vi "signal_mapping_PMT-measurement_7_9.vi"() -> ()   [LabVIEW 2024]
uses:
  <vilib>/Analysis/1siggen.llb/Ramp Pattern by Samples.vi
  <vilib>/Utility/file.llb/Write Delimited Spreadsheet (string).vi
  <vilib>/Utility/file.llb/Write Delimited Spreadsheet (DBL).vi
  <vilib>/Analysis/NI_AALBase.lvlib
panel:
  in  "max_step (V)":dbl format="%#_13g"
  in  "ChB Parameter 1":u16(ring)=2 items=["X", "Y", "R", "Theta", "Frequency", "Noise", "Xh1", "Yh1", "Rh1", "Theta h1", "Xh2", "Yh2", "Rh2", "Theta h2"]
  in  "ChB Parameter 2":u16(ring)=2 items=["X", "Y", "R", "Theta", "Frequency", "Noise", "Xh1", "Yh1", "Rh1", "Theta h1", "Xh2", "Yh2", "Rh2", "Theta h2"]
  in  "ChA Parameter 2":u16(ring)=2 items=["X", "Y", "R", "Theta", "Frequency", "Noise", "Xh1", "Yh1", "Rh1", "Theta h1", "Xh2", "Yh2", "Rh2", "Theta h2"]
  in  "ChA Parameter 1":u16(ring)=2 items=["X", "Y", "R", "Theta", "Frequency", "Noise", "Xh1", "Yh1", "Rh1", "Theta h1", "Xh2", "Yh2", "Rh2", "Theta h2"]
  in  "Set Sensitivities":bool
  in  "A Sensitivity":u16(ring)=20 items=["1 nV/fA", "2 nV/fA", "5 nV/fA", "10 nV/fA", "20 nV/fA", "50 nV/fA", "100 nV/fA", "200 nV/fA", "500 nV/fA", "1 uV/pA", "2 uV/pA", "5 uV/pA", "10 uV/pA", "20 uV/pA", "50 uV/pA", "100 uV/pA", "200 uV/pA", "500 uV/pA", "1 mV/nA", "2 mV/nA", "5 mV/nA", "10 mV/nA", "20 mV/nA", "50 mV/nA", "100 mV/nA", "200 mV/nA", "500 mV/nA", "1 V/uA"]
  in  "B Sensitivity":u16(ring)=20 items=["1 nV/fA", "2 nV/fA", "5 nV/fA", "10 nV/fA", "20 nV/fA", "50 nV/fA", "100 nV/fA", "200 nV/fA", "500 nV/fA", "1 uV/pA", "2 uV/pA", "5 uV/pA", "10 uV/pA", "20 uV/pA", "50 uV/pA", "100 uV/pA", "200 uV/pA", "500 uV/pA", "1 mV/nA", "2 mV/nA", "5 mV/nA", "10 mV/nA", "20 mV/nA", "50 mV/nA", "100 mV/nA", "200 mV/nA", "500 mV/nA", "1 V/uA"]
  in  "Lock-In Num Avgs":i32
  out "错误输出":errorcluster
  in  "OE1022D 2":refnum<visa-resource-name> caption="OE1022D"
  out "序列号":string
  in  "ms to wait after move":u32=1
  in  "ANC300 address":refnum<visa-resource-name>="COM8"
  in  "Snake":bool
  in  "File to save to":path
  in  "Select Scan Type":u16(ring)=1 items=["line scan", "rectangular scan"]
  in  "scan points":i32
  in  "y end":i32
  in  "x end":i32
  in  "y start":i32
  in  "x start":i32
  in  "y scan points":i32
  in  "x scan points":i32
  in  "y scan size":i32
  in  "x scan size":i32
  in  "y center":i32
  in  "x center":i32
  # "Scaning Setup"
  # "Rectangular Scan Parameters"
  # "Line Scan Parameters"
  # "Measurement Setup"
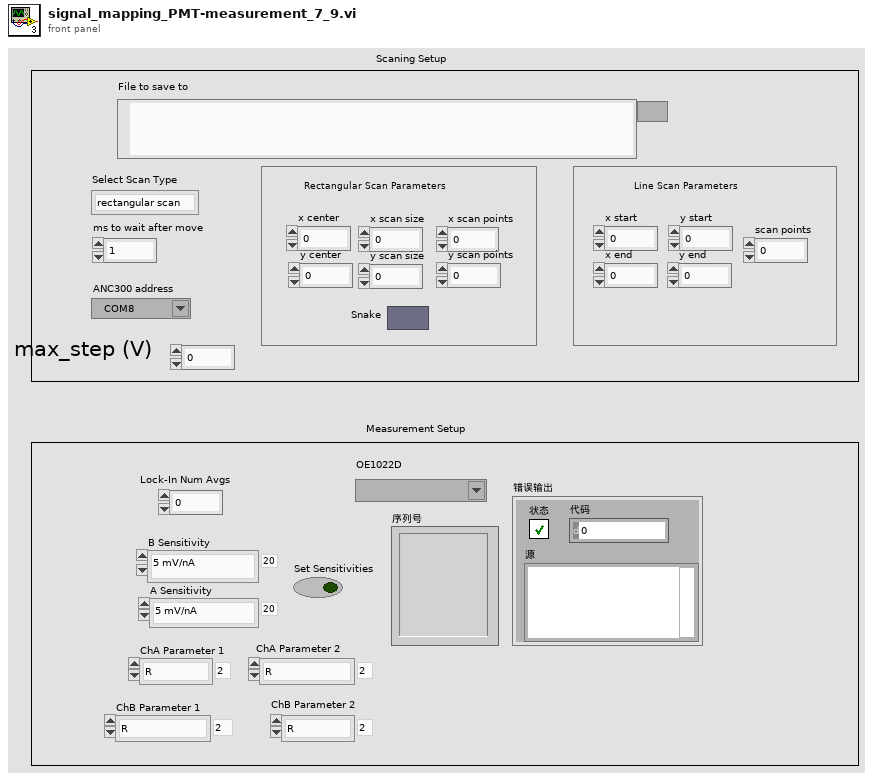
[diagram p1: front panel]
types:
  T1 = cluster{"error ":bool, "error number":i32, "error code":string}
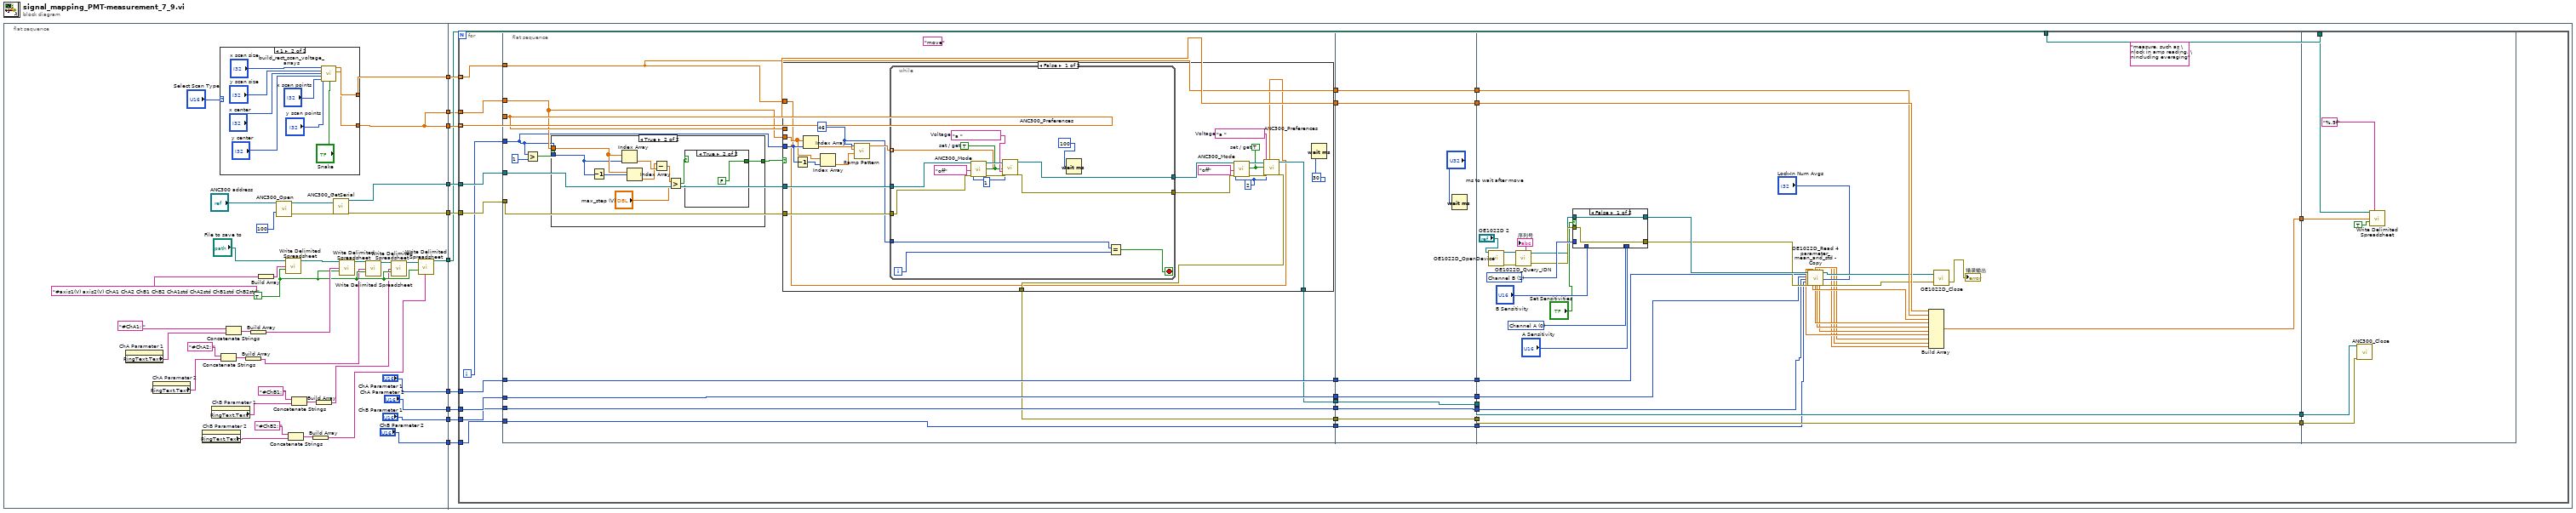
[diagram p0: block diagram]
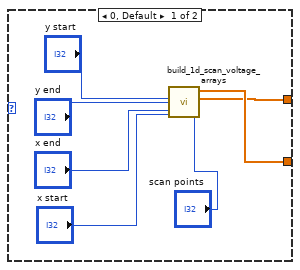
[diagram p2: hidden frame]
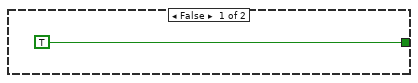
[diagram p3: hidden frame]
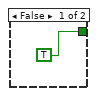
[diagram p4: hidden frame]
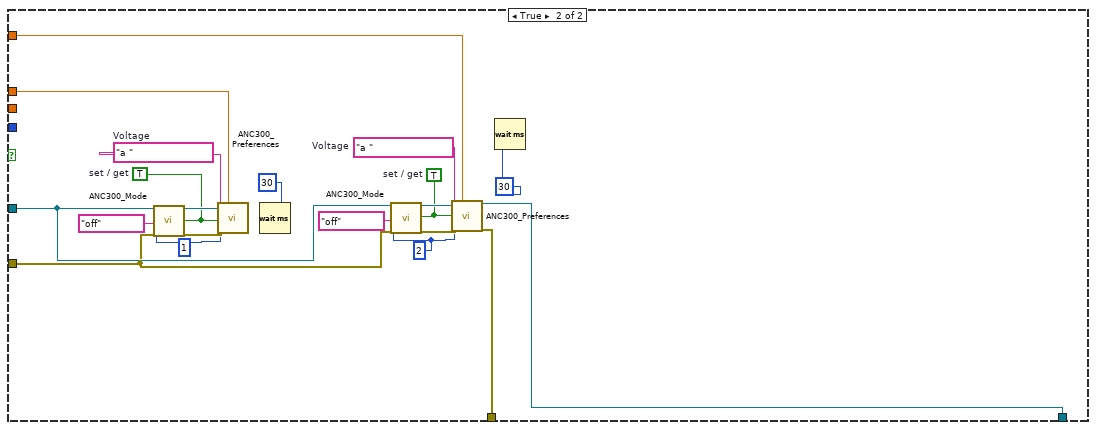
[diagram p5: hidden frame]
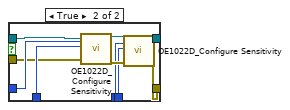
[diagram p6: hidden frame]
diagram:
  n1 = flat-sequence {
    tunnel: [w11] -> w10
    tunnel: [w48] -> w9
    tunnel: [w43] -> w8
    tunnel: [w42] -> w7
    tunnel: ["ChA Parameter 1"] -> w6
    tunnel: ["ChA Parameter 2"] -> w5
    tunnel: ["ChB Parameter 1"] -> w4
    tunnel: ["ChB Parameter 2"] -> w3
    tunnel: [w25] -> w2
    tunnel: [w11] -> w1
    tunnel: w10 -> [w74]
    tunnel: w9 -> [w73]
    tunnel: w8 -> [w72]
    tunnel: w7 -> [w71]
    tunnel: w6 -> [w69]
    tunnel: w5 -> [w68]
    tunnel: w4 -> [w67]
    tunnel: w3 -> [w66]
    tunnel: w2 -> [w70]
    tunnel: w1 -> [w65]
    frame #0 {
      w24 = TRUE
      n2 = property on="ChA Parameter 1" class="Ring (strict)"() -> ("RingText.Text"=w33:string)  [unwired: 2 in, 2 out]
      n3 = property on="ChA Parameter 2" class="Ring (strict)"() -> ("RingText.Text"=w22:string)  [unwired: 2 in, 2 out]
      n4 = property on="ChB Parameter 2" class="Ring (strict)"() -> ("RingText.Text"=w13:string)  [unwired: 2 in, 2 out]
      n5 = property on="ChB Parameter 1" class="Ring (strict)"() -> ("RingText.Text"=w12:string)  [unwired: 2 in, 2 out]
      n6 = case shown="1" "Select Scan Type" {
        tunnel: [w49 w64] -> w48
        tunnel: [w50 w63] -> w11
        frame 0, Default {
          n7 = call "build_1d_scan_voltage_arrays.vi"("y end"="y end", "y start"="y start", "scan points"="scan points", "x start"="x start", "x end"="x end") -> ("y voltage array"=w49:dbl[], "x voltage array"=w50:dbl[])  [unwired: 5 in]
        }
        frame 1 {
          n8 = call "build_rect_scan_voltage_arrays.vi"("y scan points"="y scan points", "y scan size"="y scan size", "x center"="x center", "Snake"="Snake", "y center"="y center", "x scan points"="x scan points", "x scan size"="x scan size") -> ("y voltage array"=w64:dbl[], "x voltage array"=w63:dbl[])  [unwired: 3 in]
        }
      }
      n9 = Concatenate Strings("#ChA2: ", w22) -> (w23:string)
      n10 = Concatenate Strings("#ChA1: ", w33) -> (w30:string)
      n11 = Build Array(w23) -> (w20:string[])
      n12 = Build Array(w30) -> (w29:string[])
      n13 = Build Array("#axis1(V) axis2(V) ChA1 ChA2 ChB1 ChB2 ChA1std ChA2std ChB1std ChB2std") -> (w38:string[])
      n14 = call "ANC300_Open.vi"("ANC300 Communication Port In"="ANC300 address", "milliseconds to wait"=u32 100 ("millisecond timer value")) -> ("ANC300 Communication Port Out"=w44:refnum<visa-resource-name>, "error out"=w41:T1)  [unwired: 13 in, 3 out]
      n15 = call-poly <vilib>:"Write Delimited Spreadsheet.vi"("file path (dialog if empty)"="File to save to", "1D data"=w38, "append to file? (new file:F)"=w24) -> ("new file path (Not A Path if cancelled)"=w31:path)  [unwired: 11 in, 1 out]
      n16 = Concatenate Strings("#ChB2: ", w13) -> (w17:string)
      n17 = Concatenate Strings("#ChB1: ", w12) -> (w19:string)
      n18 = Build Array(w17) -> (w15:string[])
      n19 = Build Array(w19) -> (w14:string[])
      n20 = call "ANC300_GetSerial.vi"("ANC300 Communication Port In"=w44, "error in"=w41) -> ("ANC300 Communication Port Out"=w43:refnum<visa-resource-name>, "error out"=w42:T1)  [unwired: 10 in, 6 out]
      n21 = call-poly <vilib>:"Write Delimited Spreadsheet.vi"("file path (dialog if empty)"=w31, "1D data"=w29, "append to file? (new file:F)"=w24) -> ("new file path (Not A Path if cancelled)"=w28:path)  [unwired: 11 in, 1 out]
      n22 = call-poly <vilib>:"Write Delimited Spreadsheet.vi"("file path (dialog if empty)"=w28, "1D data"=w20, "append to file? (new file:F)"=w24) -> ("new file path (Not A Path if cancelled)"=w27:path)  [unwired: 11 in, 1 out]
      n23 = call-poly <vilib>:"Write Delimited Spreadsheet.vi"("file path (dialog if empty)"=w27, "1D data"=w14, "append to file? (new file:F)"=w24) -> ("new file path (Not A Path if cancelled)"=w26:path)  [unwired: 11 in, 1 out]
      n24 = call-poly <vilib>:"Write Delimited Spreadsheet.vi"("file path (dialog if empty)"=w26, "1D data"=w15, "append to file? (new file:F)"=w24) -> ("new file path (Not A Path if cancelled)"=w25:path)  [unwired: 11 in, 1 out]
    }
    frame #1 {
      n25 = for {
        tunnel: w74 -> [w104] mode=indexing
        tunnel: w73 -> [w103] mode=indexing
        tunnel: w72 -> [w102]
        tunnel: w71 -> [w101]
        tunnel: w70 -> [w95]
        tunnel: w69 -> [w88]
        tunnel: w68 -> [w85]
        tunnel: w67 -> [w81]
        tunnel: w66 -> [w79]
        tunnel: w65 -> [w76]
        i -> [w75]
        n26 = flat-sequence {
          tunnel: w104 -> [w117]
          tunnel: w103 -> [w116]
          tunnel: w102 -> [w119]
          tunnel: w101 -> [w118]
          tunnel: [w117] -> w98
          tunnel: [w116] -> w97
          tunnel: [w105] -> w94
          tunnel: [w106] -> w91
          tunnel: w88 -> [w115]
          tunnel: [w115] -> w86
          tunnel: w85 -> [w114]
          tunnel: [w114] -> w83
          tunnel: [w113] -> w82
          tunnel: w81 -> [w113]
          tunnel: w79 -> [w112]
          tunnel: [w112] -> w77
          tunnel: w76 -> [w108]
          tunnel: w75 -> [w107]
          tunnel: [w195] -> w99
          tunnel: w98 -> [w195]
          tunnel: w97 -> [w194]
          tunnel: [w194] -> w96
          tunnel: w94 -> [w193]
          tunnel: [w193] -> w93
          tunnel: [w192] -> w92
          tunnel: w91 -> [w192]
          tunnel: [w191] -> w87
          tunnel: w86 -> [w191]
          tunnel: [w190] -> w84
          tunnel: w83 -> [w190]
          tunnel: w82 -> [w189]
          tunnel: [w189] -> w80
          tunnel: [w188] -> w78
          tunnel: w77 -> [w188]
          tunnel: [w230] -> w100
          tunnel: w99 -> [w224]
          tunnel: w96 -> [w223]
          tunnel: w93 -> [w215]
          tunnel: w92 -> [w214]
          tunnel: [w215] -> w90
          tunnel: [w214] -> w89
          tunnel: w87 -> [w200]
          tunnel: w84 -> [w199]
          tunnel: w80 -> [w198]
          tunnel: w78 -> [w197]
          tunnel: w100 -> [w247]
          tunnel: w95 -> [w245]
          tunnel: w90 -> [w244]
          tunnel: w89 -> [w243]
          frame #0 {
            (unwired) "move"
            n27 = Greater?(x=w107, y=1) -> (0:w111:bool)
            n28 = case shown="True" w111 {
              tunnel: w108 -> [_ w129]
              tunnel: w107 -> [_ w128]
              tunnel: [TRUE w121] -> w109
              frame False {
              }
              frame True {
                n29 = Decrement(x=w128) -> (x-1=w127:i32)
                n30 = Index Array(array=w129, index=w128) -> (element=w126:dbl)
                n31 = Index Array(array=w129, index=w127) -> (element=w125:dbl)
                n32 = Subtract(x=w125, y=w126) -> (x-y=w124:dbl)
                n33 = Greater?(x=w124, y="max_step (V)") -> (0:w122:bool)
                n34 = case shown="True" w122 {
                  tunnel: [TRUE FALSE] -> w121
                  frame False {
                  }
                  frame True {
                  }
                }
              }
            }
            n35 = case shown="False" w109 {
              tunnel: w119 -> [w146 w174]
              tunnel: w118 -> [w145 w173]
              tunnel: w117 -> [_ w171]
              tunnel: w116 -> [w132 w170]
              tunnel: w108 -> [w150 _]
              tunnel: w107 -> [w152 _]
              tunnel: [w134 w168] -> w106
              tunnel: [w133 w169] -> w105
              frame False {
                w138 = 2
                w139 = TRUE  # set / get
                w141 = "a "  # Voltage
                w144 = 46
                n36 = Decrement(x=w152) -> (x-1=w151:i32)
                n37 = Index Array(array=w150, index=w152) -> (element=w149:dbl)
                n38 = Index Array(array=w150, index=w151) -> (element=w148:dbl)
                n39 = call-poly <vilib>:"Ramp Pattern.vi"("start"=w148, "end"=w149, "samples"=w144) -> ("Ramp Pattern"=w147:dbl[])  [unwired: 7 in, 1 out]
                n40 = while {
                  tunnel: w147 -> [w158] mode=indexing
                  tunnel: w146 -> [w160]
                  tunnel: w145 -> [w159]
                  tunnel: w144 -> [w156]
                  tunnel: [w154] -> w136
                  tunnel: [w153] -> w135
                  i -> [w157]
                  stop <- w155 stop-if-true
                  w161 = 1
                  w162 = TRUE  # set / get
                  w165 = "a "  # Voltage
                  n41 = call "ANC300_Mode.vi"("ANC300 Communication Port In"=w160, "Axis"=w161, "axis mode in"="off", "error in"=w159, "set / get"=w162) -> ("ANC300 Communication Port Out"=w167:refnum<visa-resource-name>, "error out"=w166:T1)  [unwired: 8 in, 5 out]
                  n42 = call "ANC300_Preferences.vi"("ANC300 Communication Port In"=w167, "Axis"=w161, "value in"=w158, "parameter"=w165, "error in"=w166, "set / get"=w162) -> ("ANC300 Communication Port Out"=w154:refnum<visa-resource-name>, "error out"=w153:T1)  [unwired: 6 in, 6 out]
                  n43 = Wait (ms)(milliseconds to wait=u32 100 ("1: ms to wait")) -> ()  [unwired: 1 out]
                  n44 = Equal?(x=w156, y=w157) -> (x = y?=w155:bool)
                }
                n45 = call "ANC300_Mode.vi"("ANC300 Communication Port In"=w136, "Axis"=w138, "axis mode in"="off", "error in"=w135, "set / get"=w139) -> ("ANC300 Communication Port Out"=w143:refnum<visa-resource-name>, "error out"=w142:T1)  [unwired: 8 in, 5 out]
                n46 = call "ANC300_Preferences.vi"("ANC300 Communication Port In"=w143, "Axis"=w138, "value in"=w132, "parameter"=w141, "error in"=w142, "set / get"=w139) -> ("ANC300 Communication Port Out"=w133:refnum<visa-resource-name>, "error out"=w134:T1)  [unwired: 6 in, 6 out]
                n47 = Wait (ms)(milliseconds to wait=u32 30 ("2: ms to wait")) -> ()  [unwired: 1 out]
              }
              frame True {
                w175 = 2
                w176 = 1
                w177 = TRUE  # set / get
                w179 = "a "  # Voltage
                w182 = TRUE  # set / get
                w185 = "a "  # Voltage
                n48 = call "ANC300_Mode.vi"("ANC300 Communication Port In"=w174, "Axis"=w176, "axis mode in"="off", "error in"=w173, "set / get"=w182) -> ("ANC300 Communication Port Out"=w187:refnum<visa-resource-name>, "error out"=w186:T1)  [unwired: 8 in, 5 out]
                n49 = call "ANC300_Preferences.vi"("ANC300 Communication Port In"=w187, "Axis"=w176, "value in"=w171, "parameter"=w185, "error in"=w186, "set / get"=w182) -> ()  [unwired: 6 in, 8 out]
                n50 = Wait (ms)(milliseconds to wait=u32 30 ("1: ms to wait")) -> ()  [unwired: 1 out]
                n51 = call "ANC300_Mode.vi"("ANC300 Communication Port In"=w174, "Axis"=w175, "axis mode in"="off", "error in"=w173, "set / get"=w177) -> ("ANC300 Communication Port Out"=w181:refnum<visa-resource-name>, "error out"=w180:T1)  [unwired: 8 in, 5 out]
                n52 = call "ANC300_Preferences.vi"("ANC300 Communication Port In"=w181, "Axis"=w175, "value in"=w170, "parameter"=w179, "error in"=w180, "set / get"=w177) -> ("ANC300 Communication Port Out"=w169:refnum<visa-resource-name>, "error out"=w168:T1)  [unwired: 6 in, 6 out]
                n53 = Wait (ms)(milliseconds to wait=u32 30 ("2: ms to wait")) -> ()  [unwired: 1 out]
              }
            }
          }
          frame #1 {
            n54 = Wait (ms)(milliseconds to wait="ms to wait after move") -> ()  [unwired: 1 out]
          }
          frame #2 {
            w218 = u8 0 items=["Channel A", "Channel B"] ("OE1022D A/B")
            w222 = u8 1 items=["Channel A", "Channel B"] ("OE1022D A/B")
            (unwired) "measure, such as \nlock in amp reading, \nincluding everaging"
            n55 = call "OE1022D_OpenDevice.vi"("VISA resource name"="OE1022D 2") -> ("VISA资源名称输出"=w227:refnum<visa-resource-name>, "错误输出"=w228:errorcluster)  [unwired: 17 in]
            n56 = call "OE1022D_Query_IDN.vi"("错误输入（无错误）"=w228, "VISA resource name"=w227) -> ("错误输出"=w220:errorcluster, "序列号"=→"序列号":string, "VISA resource name out"=w219:refnum<visa-resource-name>)  [unwired: 1 in]
            n57 = case shown="False" "Set Sensitivities" {
              tunnel: w222 -> [_ w242]
              tunnel: "B Sensitivity" -> [_ w241]
              tunnel: w220 -> [w231 w240]
              tunnel: w219 -> [w232 w239]
              tunnel: [w232 w236] -> w213
              tunnel: [w231 w235] -> w212
              tunnel: w218 -> [_ w234]
              tunnel: "A Sensitivity" -> [_ w233]
              frame False {
              }
              frame True {
                n58 = call "OE1022D_Configure Sensitivity.vi"("VISA resource name"=w239, "OE1022D A/B"=w242, "Sensitivity"=w241, "error in (no error)"=w240) -> ("VISA resource name out"=w237:refnum<visa-resource-name>, "error out"=w238:errorcluster)  [unwired: 14 in]
                n59 = call "OE1022D_Configure Sensitivity.vi"("VISA resource name"=w237, "OE1022D A/B"=w234, "Sensitivity"=w233, "error in (no error)"=w238) -> ("VISA resource name out"=w236:refnum<visa-resource-name>, "error out"=w235:errorcluster)  [unwired: 14 in]
              }
            }
            n60 = call "OE1022D_Read 4 parameter_mean_and_std - Copy.vi"("VISA resource name"=w213, "ChA Parameter 1"=w200, "ChA Parameter 2"=w199, "ChB Parameter 1"=w198, "ChB Parameter 2"=w197, "错误输入（无错误）"=w212, "Num Averages"="Lock-In Num Avgs") -> ("Measurement STD"=w204:dbl, "Measurement"=w208:dbl, "Measurement STD 2"=w203:dbl, "Measurement 2"=w207:dbl, "Measurement STD 3"=w202:dbl, "Measurement 3"=w206:dbl, "Measurement STD 4"=w201:dbl, "Measurement 4"=w205:dbl, "VISA resource name out"=w210:refnum<visa-resource-name>, "error out"=w211:errorcluster)  [unwired: 3 in]
            n61 = Build Array(w224, w223, w208, w207, w206, w205, w204, w203, w202, w201) -> (w230:dbl[])
            n62 = call "OE1022D_Close.vi"("错误输入（无错误）"=w211, "VISA resource name"=w210) -> ("错误输出"=→"错误输出":errorcluster)  [unwired: 1 in]
          }
          frame #3 {
            n63 = call "ANC300_Close.vi"("ANC300 Communication Port In"=w244, "error in"=w243) -> ()  [unwired: 17 in, 1 out]
            n64 = call-poly <vilib>:"Write Delimited Spreadsheet.vi"("file path (dialog if empty)"=w245, "format (%.3f)"="%.9f", "1D data"=w247, "append to file? (new file:F)"=TRUE) -> ()  [unwired: 10 in, 2 out]
          }
        }
      }
    }
  }
